vi "Valid Measurement Service Name.vi"(8 "error in":errorcluster, 10 "Valid Service Name":string, 11 "Project ref":refnum<vi>) -> (0 "error out":errorcluster, 3 "Valid Name?":bool)   [LabVIEW 2020, in "MeasurementService Editor.lvlib"]
uses:
  MeasurementService Editor.lvlib
  48953c88-0603-4c13-ba6a-df914321b09e.vi
  4e5bfea7-4973-4dbf-a6b2-c9d09f62e007.vi
  <vilib>/Comparison/Equal/Equal Functor/Equal Functor.lvclass
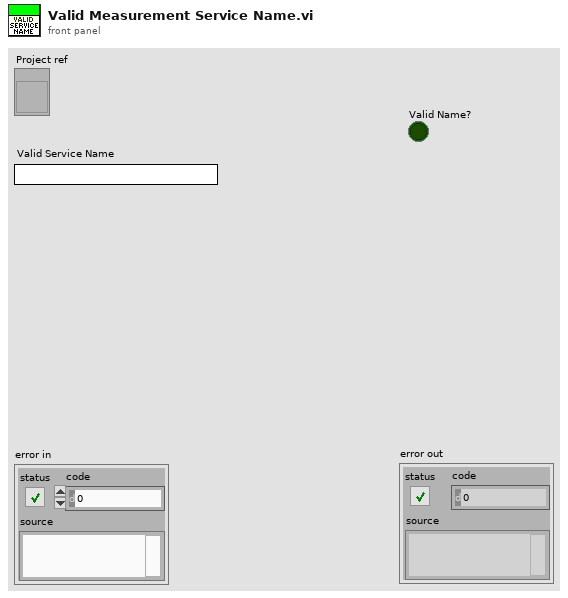
[diagram p1: front panel]
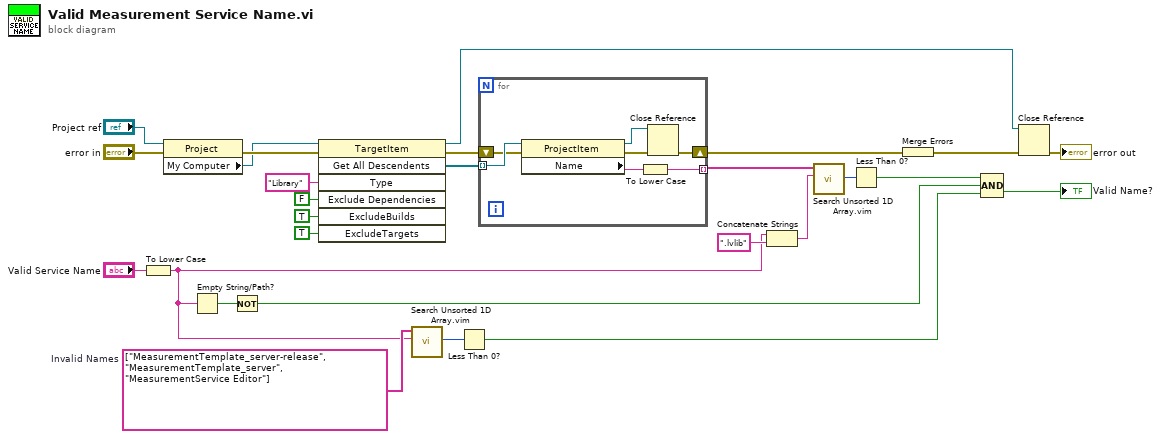
[diagram p0: block diagram]
diagram:
  w4 = string[] ["MeasurementTemplate_server-release", "MeasurementTemplate_server", "MeasurementService Editor"]  # Invalid Names
  n1 = To Lower Case(string="Valid Service Name") -> (all lower case string=w3:string)
  n2 = property class="Project"(reference="Project ref", error in="error in") -> (error out=w11:errorcluster, "My Computer"=w8:refnum<vi>)  [unwired: 1 out]
  n3 = Empty String/Path?(string/path=w3) -> (empty?=w6:bool)
  n4 = Not(x=w6) -> (.not. x?=w5:bool)
  n5 = invoke class="TargetItem" method="Get All Descendents"(reference=w8, error in=w11, "Type"="Library", "Exclude Dependencies"=FALSE ("ExcludeDependencies"), "ExcludeBuilds"=TRUE, "ExcludeTargets"=TRUE) -> (reference out=w16:refnum<vi>, error out=w18:errorcluster, "All Descendents"=w23:refnum<vi>[])  [unwired: 1 in, 4 out]
  n6 = call "Search Unsorted 1D Array.vim"("element"=w3, "unsorted 1D array"=w4) -> ("index of element"=w2:i32)  [unwired: 9 in]
  n7 = Less Than 0?(x=w2) -> (x < 0?=w1:bool)
  n8 = for {
    tunnel: w23 -> [w34] mode=indexing
    tunnel: [w28] -> w22 mode=indexing
    shift-right: [w30] -> w17
    shift-left: w18 -> [w32]
    n9 = property class="ProjectItem"(reference=w34, error in=w32) -> (reference out=w29:refnum<vi>, error out=w31:errorcluster, "Name"=w33:string)
    n10 = To Lower Case(string=w33) -> (all lower case string=w28:string)
    n11 = Close Reference(reference=w29, error in (no error)=w31) -> (error out=w30:errorcluster)
  }
  n12 = Concatenate Strings(w3, ".lvlib" ("string")) -> (w13:string)
  n13 = call "Search Unsorted 1D Array.vim"("element"=w13, "unsorted 1D array"=w22) -> ("index of element"=w21:i32)  [unwired: 9 in]
  n14 = Less Than 0?(x=w21) -> (x < 0?=w20:bool)
  n15 = Merge Errors(w17) -> (w7:errorcluster)
  n16 = Compound Arithmetic op=AND(w20, w5, w1) -> (→"Valid Name?":bool)
  n17 = Close Reference(reference=w16, error in (no error)=w7) -> (error out=→"error out":errorcluster)
